vi "Periodic Tasks.vi"(8 "error in":errorcluster) -> ()   [LabVIEW 2018]
doc: "This VI runs in parallel to other tasks. It can contain as many user-defined periodic loops as you need. These can carry out PID or other sorts of timed response."
uses:
  <vilib>/Rock Robotics/WPI/Solenoid/WPI_SolenoidValue.ctl
  <vilib>/Rock Robotics/WPI/ThirdParty/Phoenix-LabVIEW/Motor Controller/Controls/CTRE_Phoenix_MotorControl_ControlMode.ctl
  <vilib>/Rock Robotics/WPI/Utilities/WPI_GetSetVariantRefNum.vi
  Robot Global Data.vi
  <vilib>/Rock Robotics/Network Tables/NT Write Boolean.vi
  <vilib>/Rock Robotics/WPI/ThirdParty/Phoenix-LabVIEW/Motor Controller/Get/CTRE_Phoenix_MotorController_GetSelectedSensorData.vi
  <vilib>/Rock Robotics/Network Tables/NT Write Number.vi
  <vilib>/Rock Robotics/WPI/ThirdParty/Phoenix-LabVIEW/Motor Controller/Get/CTRE_Phoenix_MotorController_GetGeneralStatus.vi
  <vilib>/Rock Robotics/WPI/ThirdParty/Phoenix-LabVIEW/Motor Controller/Get/CTRE_Phoenix_MotorController_GetOutputCurrent_Enhanced.vi
  <vilib>/Rock Robotics/WPI/Solenoid/WPI_SolenoidSetEnum.vi
  Intake Constants.vi
  Elevator Constants.vi
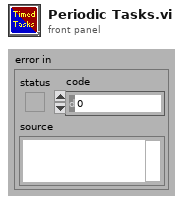
[diagram p1: front panel]
types:
  T1 = enum16{"Zero Power", "Push Cargo", "Pull Cargo", "Hold Cargo"}
  T2 = enum16{"In Up Position", "Seek Up Stage 1", "Seek Up Stage 2", "Seek Normally", "Test Enabled"}
  T3 = typedef "WPI_MotorControlDeviceRef.ctl" = cluster{"DeviceStatus":errorcluster, "Type":T4, "PWM":cluster{"PWM Channel":T5, "DeadBand":T6}, "CAN":cluster{"Device Number":u8, "SetOutput VI Ref":variant, "GetOutput VI Ref":variant, "Enable VI Ref":variant, "Disable VI Ref":variant, "Data":variant}, "Invert":bool, "DIO PWM":cluster{"PWM \"Enable\" Channel":T5, "DIOChannel":T7, "PWM Rate":dbl}}
  T4 = typedef "WPI_MotorControlType.ctl" = enum16{"PWM", "CAN", "DIO PWM"}
  T5 = typedef "FPGA_DIOPWMChannel.ctl" = enum8{"PWM 0", "PWM 1", "PWM 2", "PWM 3", "PWM 4", "PWM 5", "PWM 6", "PWM 7", "PWM 8", "PWM 9", "PWM MXP 0", "PWM MXP 1", "PWM MXP 2", "PWM MXP 3", "PWM MXP 4", "PWM MXP 5", "PWM MXP 6", "PWM MXP 7", "PWM MXP 8", "PWM MXP 9", "Invalid"}
  T6 = typedef "WPI_PWMDeadband.ctl" = cluster{"Name":string, "maxPositivePwm":i32, "minPositivePwm":i32, "centerPwm":i32, "maxNegativePwm":i32, "minNegativePwm":i32, "angularRange":u16}
  T7 = typedef "FPGA_DIOChannel.ctl" = enum8{"DIO 0", "DIO 1", "DIO 2", "DIO 3", "DIO 4", "DIO 5", "DIO 6", "DIO 7", "DIO 8", "DIO 9", "DIO MXP 0", "DIO MXP 1", "DIO MXP 2", "DIO MXP 3", "DIO MXP 4", "DIO MXP 5", "DIO MXP 6", "DIO MXP 7", "DIO MXP 8", "DIO MXP 9", "DIO MXP 10", "DIO MXP 11", "DIO MXP 12", "DIO MXP 13", "DIO MXP 14", "DIO MXP 15", "SPI Port CS1", "SPI Port CS2", "SPI Port CS3", "SPI Port MISO", "SPI Port MOSI", "Invalid"}
  T8 = typedef "WPI_JoystickDevRef.ctl" = cluster{"Device":T9}
  T9 = typedef "WPI_JoystickDeviceEnum.ctl" = enum16{"USB 0", "USB 1", "USB 2", "USB 3", "USB 4", "USB 5"}
  T10 = typedef "WPI_RobotDriveDevRef.ctl" = cluster{"DevStatus":errorcluster, "Motors[]":T3[], "Square Inputs":bool, "Max Output":dbl}
  T11 = typedef "WPI_SolenoidDevRef.ctl" = cluster{"DevStatus":errorcluster, "Pneumatics Control Module":u8, "Forward Solenoid Channel":T12, "Reverse Solenoid Channel":T12}
  T12 = typedef "WPI_SolenoidChannel.ctl" = enum8{"Solenoid 0", "Solenoid 1", "Solenoid 2", "Solenoid 3", "Solenoid 4", "Solenoid 5", "Solenoid 6", "Solenoid 7", "Invalid"}
  T13 = typedef "WPI_CompressorDevRef.ctl" = cluster{"DevStatus":errorcluster, "Pneumatics Control Module":u8}
  T14 = cluster{"PhoenixMotorControlDevRef":T3, "PhoenixMotorControlDevRef":T3, "PhoenixMotorControlDevRef":T3}
  T15 = cluster{"JoystickDevRef":T8, "RobotDriveDevRef":T10, "SolenoidDevRef":T11, "SolenoidDevRef":T11, "CompressorDevRef":T13, "JoystickDevRef":T8}
  T16 = typedef "CTRE_Phoenix_MotorControl_ControlMode.ctl" = u16
  T17 = typedef "WPI_SolenoidValue.ctl" = enum16{"Off", "On", "Forward", "Reverse"}
  T18 = enum16{"In Up Position", "Seek Up Stage 1", "Seek Up Stage 2", "Seek Normally"}
  T19 = typedef "WPI_DriverStationRobotMode2.ctl" = enum16{"Autonomous Disabled", "Autonomous Enabled", "Teleop Disabled", "Teleop Enabled", "Disconnected", "Finish", "Test Disabled", "Test Enabled", "Emergency Stopped"}
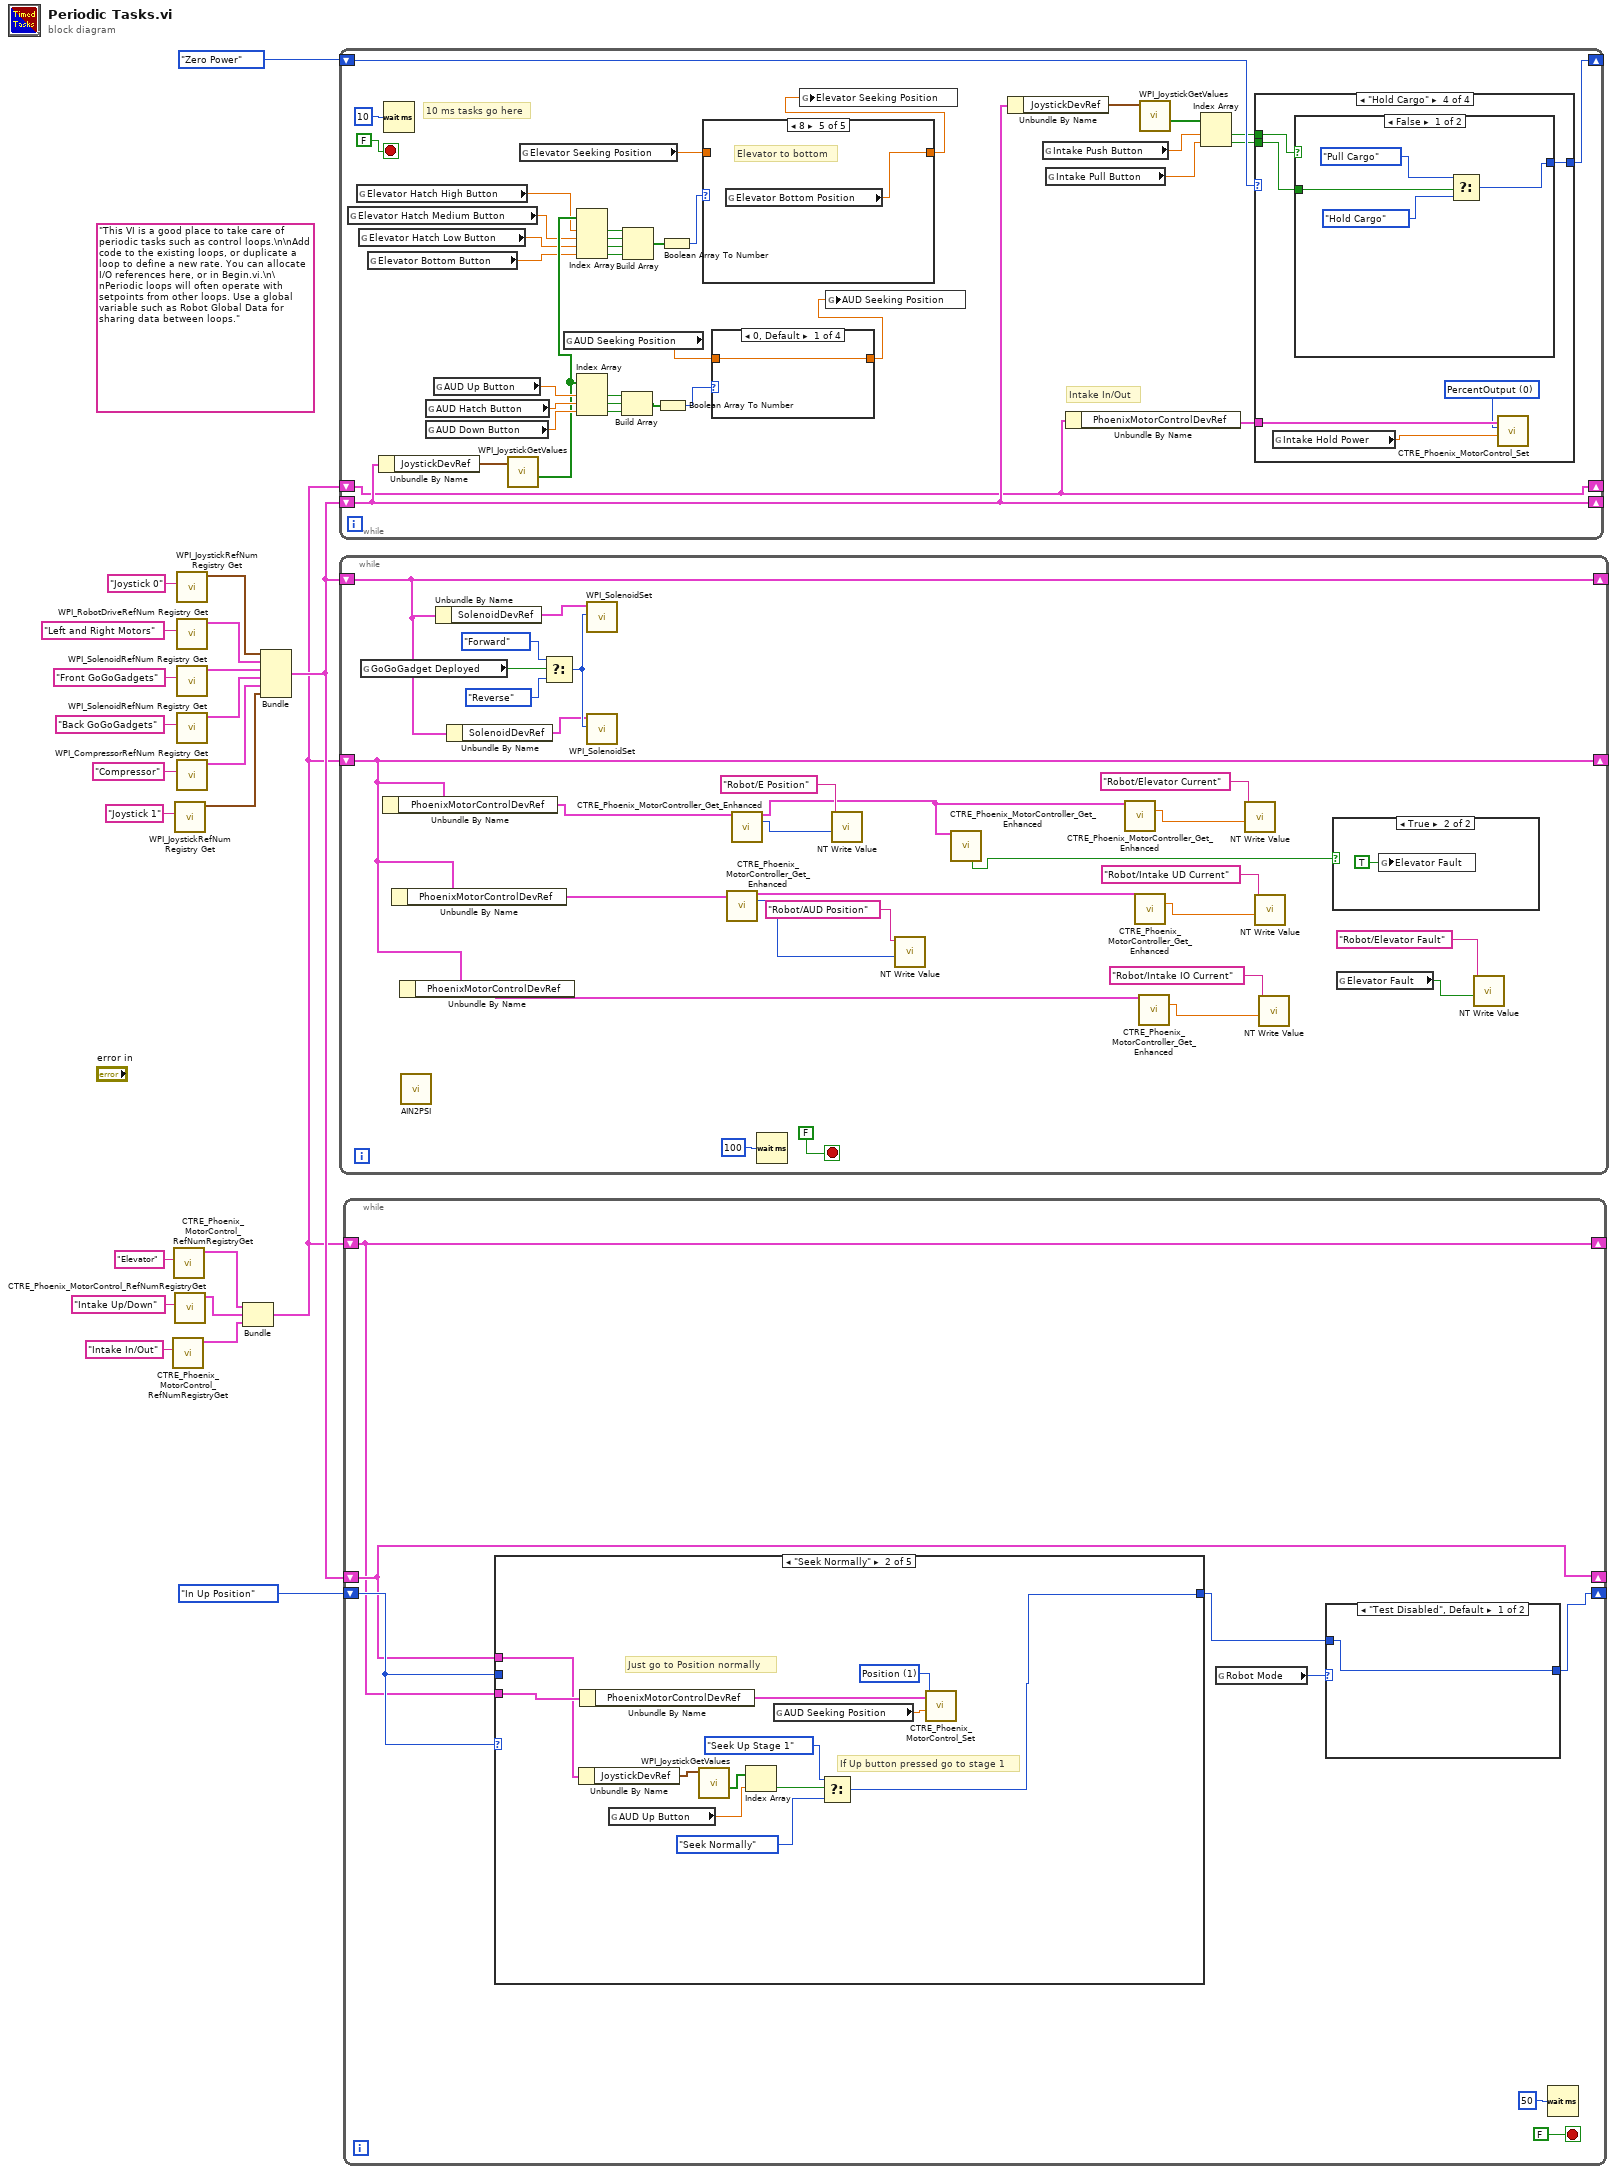
[diagram p0: block diagram]
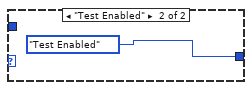
[diagram p2: hidden frame]
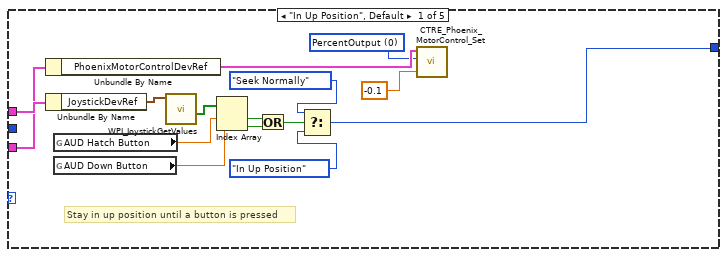
[diagram p3: hidden frame]
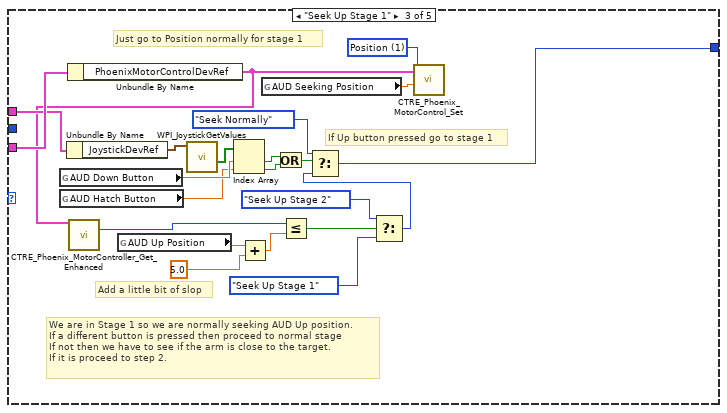
[diagram p4: hidden frame]
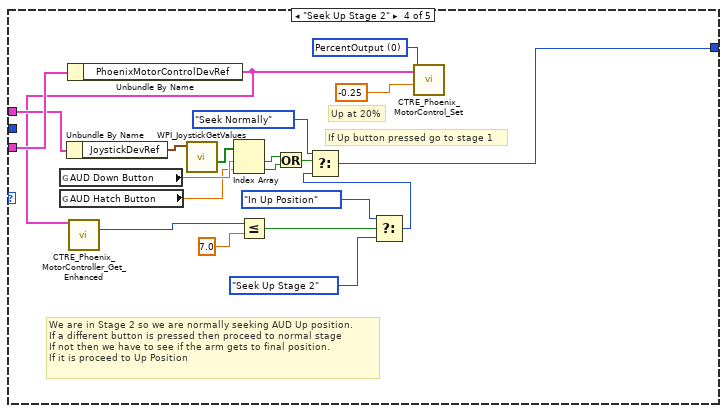
[diagram p5: hidden frame]
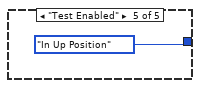
[diagram p6: hidden frame]
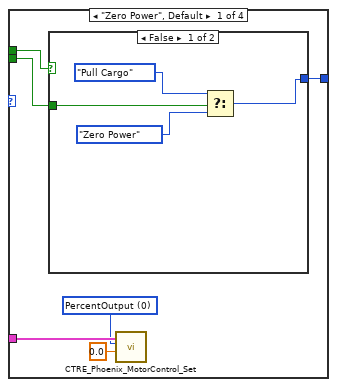
[diagram p8: hidden frame]
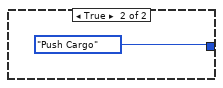
[diagram p9: hidden frame]
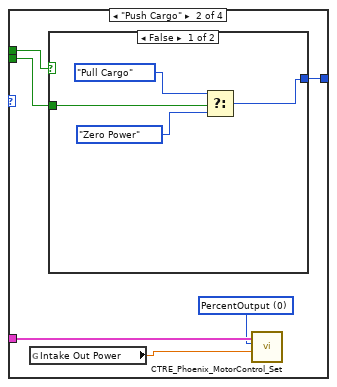
[diagram p10: hidden frame]
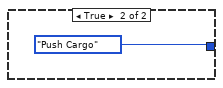
[diagram p11: hidden frame]
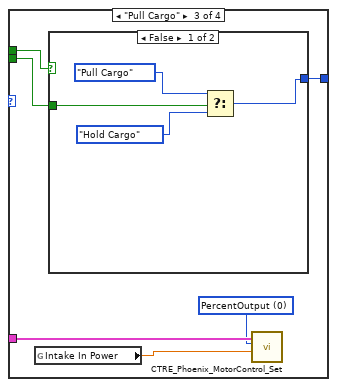
[diagram p12: hidden frame]
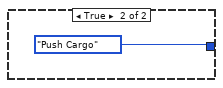
[diagram p13: hidden frame]
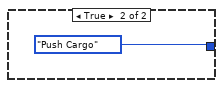
[diagram p14: hidden frame]
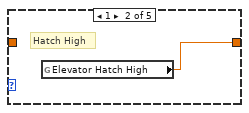
[diagram p16: hidden frame]
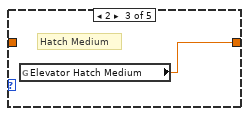
[diagram p17: hidden frame]
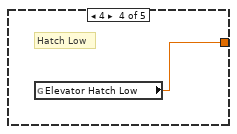
[diagram p18: hidden frame]
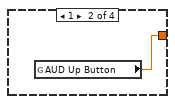
[diagram p19: hidden frame]
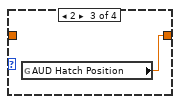
[diagram p20: hidden frame]
diagram:
  (unwired) "This VI is a good place to take care of periodic tasks such as control loops.\n\nAdd code to the existing loops, or duplicate a loop to define a new rate. You can allocate I/O references here, or in Begin.vi.\n\nPeriodic loops will often operate with setpoints from other loops. Use a global variable such as Robot Global Data for sharing data between loops."
  n1 = call <vilib>:"CTRE_Phoenix_MotorControl_RefNumRegistryGet.vi"("refnum name"="Intake In/Out") -> ("PhoenixMotorControlDevRef"=w7:T3)  [unwired: 9 in, 1 out]
  n2 = call <vilib>:"CTRE_Phoenix_MotorControl_RefNumRegistryGet.vi"("refnum name"="Elevator") -> ("PhoenixMotorControlDevRef"=w5:T3)  [unwired: 9 in, 1 out]
  n3 = call <vilib>:"WPI_JoystickRefNum Registry Get.vi"("refnum name"="Joystick 1") -> ("JoystickDevRef"=w11:T8)  [unwired: 1 in, 9 out]
  n4 = call <vilib>:"CTRE_Phoenix_MotorControl_RefNumRegistryGet.vi"("refnum name"="Intake Up/Down") -> ("PhoenixMotorControlDevRef"=w6:T3)  [unwired: 9 in, 1 out]
  n5 = call <vilib>:"WPI_JoystickRefNum Registry Get.vi"("refnum name"="Joystick 0") -> ("JoystickDevRef"=w20:T8)  [unwired: 1 in, 9 out]
  n6 = call <vilib>:"WPI_RobotDriveRefNum Registry Get.vi"("refnum name"="Left and Right Motors") -> ("RobotDriveDevRef"=w19:T10)  [unwired: 1 in, 9 out]
  n7 = call <vilib>:"WPI_SolenoidRefNum Registry Get.vi"("refnum name"="Front GoGoGadgets") -> ("SolenoidDevRef"=w18:T11)  [unwired: 9 in, 1 out]
  n8 = call <vilib>:"WPI_SolenoidRefNum Registry Get.vi"("refnum name"="Back GoGoGadgets") -> ("SolenoidDevRef"=w17:T11)  [unwired: 9 in, 1 out]
  n9 = call <vilib>:"WPI_CompressorRefNum Registry Get.vi"("refnum name"="Compressor") -> ("CompressorDevRef"=w13:T13)  [unwired: 9 in, 1 out]
  n10 = Bundle("PhoenixMotorControlDevRef"=w5, "PhoenixMotorControlDevRef"=w6, "PhoenixMotorControlDevRef"=w7) -> (w1:T14)  [unwired: 1 in]
  n11 = Bundle("JoystickDevRef"=w20, "RobotDriveDevRef"=w19, "SolenoidDevRef"=w18, "SolenoidDevRef"=w17, "CompressorDevRef"=w13, "JoystickDevRef"=w11) -> (w3:T15)  [unwired: 1 out]
  n12 = while {
    shift-right: [w32] -> _
    shift-left: w3 -> [w32]
    shift-right: [w23] -> _
    shift-left: T1."Zero Power" -> [w28]
    shift-right: [w27] -> _
    shift-left: w1 -> [w27]
    stop <- FALSE stop-if-true
    # "Intake In/Out"
    # "10 ms tasks go here"
    n13 = global read "Elevator Constants.vi" "Elevator Hatch Medium Button"() -> (w43:dbl)
    n14 = global read "Elevator Constants.vi" "Elevator Hatch High Button"() -> (w42:dbl)
    n15 = global read "Elevator Constants.vi" "Elevator Hatch Low Button"() -> (w44:dbl)
    n16 = global read "Elevator Constants.vi" "Elevator Bottom Button"() -> (w45:dbl)
    n17 = Unbundle By Name(w32) -> ("JoystickDevRef"=w57:T8)
    n18 = Wait (ms)(milliseconds to wait=u32 10) -> ()  [unwired: 1 out]
    n19 = global read "Intake Constants.vi" "AUD Hatch Button"() -> (w55:dbl)
    n20 = global read "Intake Constants.vi" "AUD Down Button"() -> (w51:dbl)
    n21 = global read "Intake Constants.vi" "AUD Up Button"() -> (w56:dbl)
    n22 = call <vilib>:"WPI_JoystickGetValues.vi"("JoystickDevRef"=w57) -> ("Buttons"=w46:bool[])  [unwired: 6 in, 4 out]
    n23 = global read "Elevator Constants.vi" "Elevator Seeking Position"() -> (w35:dbl)
    n24 = global read "Intake Constants.vi" "AUD Seeking Position"() -> (w49:dbl)
    n25 = Index Array(array=w46, index #1=w42, index #2=w43, index #3=w44, index #4=w45) -> (element #1=w38:bool, element #2=w41:bool, element #3=w39:bool, element #4=w40:bool)
    n26 = Index Array(array=w46, index #1=w56, index #2=w55, index #3=w51) -> (element #1=w54:bool, element #2=w53:bool, element #3=w52:bool)
    n27 = Build Array(w54, w53, w52) -> (w50:bool[])
    n28 = Build Array(w38, w41, w39, w40) -> (w37:bool[])
    n29 = Boolean Array To Number(Boolean array=w50) -> (number=w48:u32)
    n30 = Boolean Array To Number(Boolean array=w37) -> (number=w36:u32)
    n31 = case shown="8" w36 {
      tunnel: w35 -> [w104 _ _ _ _]
      tunnel: [w104 w105 w106 w107 w108] -> w34
      frame 0, Default {
      }
      frame 1 {
        # "Hatch High"
        n32 = global read "Elevator Constants.vi" "Elevator Hatch High"() -> (w105:dbl)
      }
      frame 2 {
        # "Hatch Medium"
        n33 = global read "Elevator Constants.vi" "Elevator Hatch Medium"() -> (w106:dbl)
      }
      frame 4 {
        # "Hatch Low"
        n34 = global read "Elevator Constants.vi" "Elevator Hatch Low"() -> (w107:dbl)
      }
      frame 8 {
        # "Elevator to bottom"
        n35 = global read "Elevator Constants.vi" "Elevator Bottom Position"() -> (w108:dbl)
      }
    }
    n36 = case shown="0, Default" w48 {
      tunnel: w49 -> [w109 _ _ _]
      tunnel: [w109 w110 w111 w112] -> w47
      frame 0, Default {
      }
      frame 1 {
        n37 = global read "Intake Constants.vi" "AUD Up Button"() -> (w110:dbl)
      }
      frame 2 {
        n38 = global read "Intake Constants.vi" "AUD Hatch Position"() -> (w111:dbl)
      }
      frame 4 {
        n39 = global read "Intake Constants.vi" "AUD Down Position"() -> (w112:dbl)
      }
    }
    n40 = global write "Elevator Constants.vi" "Elevator Seeking Position"(w34) -> ()
    n41 = global write "Intake Constants.vi" "AUD Seeking Position"(w47) -> ()
    n42 = Unbundle By Name(w32) -> ("JoystickDevRef"=w33:T8)
    n43 = global read "Intake Constants.vi" "Intake Push Button"() -> (w30:dbl)
    n44 = global read "Intake Constants.vi" "Intake Pull Button"() -> (w29:dbl)
    n45 = Unbundle By Name(w27) -> ("PhoenixMotorControlDevRef"=w26:T3)
    n46 = call <vilib>:"WPI_JoystickGetValues.vi"("JoystickDevRef"=w33) -> ("Buttons"=w31:bool[])  [unwired: 6 in, 4 out]
    n47 = Index Array(array=w31, index #1=w30, index #2=w29) -> (element #1=w25:bool, element #2=w24:bool)
    n48 = case shown="\"Hold Cargo\"" w28 {
      tunnel: w26 -> [w65 w76 w87 w98]
      tunnel: w25 -> [w62 w74 w85 w96]
      tunnel: w24 -> [w61 w73 w84 w95]
      tunnel: [w60 w72 w83 w94] -> w23
      frame "Zero Power", Default {
        w64 = T16 0 items=["PercentOutput"=0, "Position"=1, "Velocity"=2, "Current"=3, "Follower"=5, "MotionProfile"=6, "MotionMagic"=7, "MotionProfileArc"=10, "Disabled"=15] ("Control Mode")
        n49 = case shown="False" w62 {
          tunnel: w61 -> [w69 _]
          tunnel: [w66 T1."Push Cargo"] -> w60
          frame False {
            n50 = Select(t=T1."Pull Cargo", s=w69, f=T1."Zero Power") -> (s? t:f=w66:T1)
          }
          frame True {
          }
        }
        n51 = call <vilib>:"CTRE_Phoenix_MotorControl_Set.vi"("Output"=0.0, "Control Mode"=w64, "PhoenixMotorControlDevRef"=w65) -> ()  [unwired: 7 in, 2 out]
      }
      frame "Push Cargo" {
        w75 = T16 0 items=["PercentOutput"=0, "Position"=1, "Velocity"=2, "Current"=3, "Follower"=5, "MotionProfile"=6, "MotionMagic"=7, "MotionProfileArc"=10, "Disabled"=15] ("Control Mode")
        n52 = global read "Intake Constants.vi" "Intake Out Power"() -> (w71:dbl)
        n53 = case shown="False" w74 {
          tunnel: w73 -> [w80 _]
          tunnel: [w77 T1."Push Cargo"] -> w72
          frame False {
            n54 = Select(t=T1."Pull Cargo", s=w80, f=T1."Zero Power") -> (s? t:f=w77:T1)
          }
          frame True {
          }
        }
        n55 = call <vilib>:"CTRE_Phoenix_MotorControl_Set.vi"("Output"=w71, "Control Mode"=w75, "PhoenixMotorControlDevRef"=w76) -> ()  [unwired: 7 in, 2 out]
      }
      frame "Pull Cargo" {
        w86 = T16 0 items=["PercentOutput"=0, "Position"=1, "Velocity"=2, "Current"=3, "Follower"=5, "MotionProfile"=6, "MotionMagic"=7, "MotionProfileArc"=10, "Disabled"=15] ("Control Mode")
        n56 = global read "Intake Constants.vi" "Intake In Power"() -> (w82:dbl)
        n57 = case shown="False" w85 {
          tunnel: w84 -> [w91 _]
          tunnel: [w88 T1."Push Cargo"] -> w83
          frame False {
            n58 = Select(t=T1."Pull Cargo", s=w91, f=T1."Hold Cargo") -> (s? t:f=w88:T1)
          }
          frame True {
          }
        }
        n59 = call <vilib>:"CTRE_Phoenix_MotorControl_Set.vi"("Output"=w82, "Control Mode"=w86, "PhoenixMotorControlDevRef"=w87) -> ()  [unwired: 7 in, 2 out]
      }
      frame "Hold Cargo" {
        w97 = T16 0 items=["PercentOutput"=0, "Position"=1, "Velocity"=2, "Current"=3, "Follower"=5, "MotionProfile"=6, "MotionMagic"=7, "MotionProfileArc"=10, "Disabled"=15] ("Control Mode")
        n60 = global read "Intake Constants.vi" "Intake Hold Power"() -> (w93:dbl)
        n61 = case shown="False" w96 {
          tunnel: w95 -> [w102 _]
          tunnel: [w99 T1."Push Cargo"] -> w94
          frame False {
            n62 = Select(t=T1."Pull Cargo", s=w102, f=T1."Hold Cargo") -> (s? t:f=w99:T1)
          }
          frame True {
          }
        }
        n63 = call <vilib>:"CTRE_Phoenix_MotorControl_Set.vi"("Output"=w93, "Control Mode"=w97, "PhoenixMotorControlDevRef"=w98) -> ()  [unwired: 7 in, 2 out]
      }
    }
  }
  n64 = while {
    shift-right: [w132] -> _
    shift-left: w3 -> [w132]
    shift-right: [w117] -> _
    shift-left: w1 -> [w117]
    stop <- FALSE stop-if-true
    n65 = global read "Robot Global Data.vi" "GoGoGadget Deployed"() -> (w135:bool)
    n66 = Unbundle By Name(w117) -> ("PhoenixMotorControlDevRef"=w124:T3)
    n67 = Unbundle By Name(w117) -> ("PhoenixMotorControlDevRef"=w123:T3)
    n68 = Unbundle By Name(w117) -> ("PhoenixMotorControlDevRef"=w127:T3)
    n69 = call "AIN2PSI.vi"() -> ()  [unwired: 11 in, 1 out]
    n70 = Unbundle By Name(w132) -> ("SolenoidDevRef"=w134:T11)
    n71 = Unbundle By Name(w132) -> ("SolenoidDevRef"=w133:T11)
    n72 = Select(t=WPI_SolenoidValue."Forward" ("Value"), s=w135, f=WPI_SolenoidValue."Reverse") -> (s? t:f=w138:T17)
    n73 = call-poly <vilib>:"WPI_SolenoidSet.vi"("Value"=w138, "SolenoidDevRef"=w134) -> ()  [unwired: 8 in, 2 out]
    n74 = call-poly <vilib>:"WPI_SolenoidSet.vi"("Value"=w138, "SolenoidDevRef"=w133) -> ()  [unwired: 8 in, 2 out]
    n75 = call-poly <vilib>:"CTRE_Phoenix_MotorController_Get_Enhanced.vi"("PhoenixMotorControlDevRef"=w123) -> ("PhoenixMotorControlDevRef"=w122:T3, "Position (Raw Sensor Units)"=w118:i32)  [unwired: 11 in, 2 out]
    n76 = call-poly <vilib>:"CTRE_Phoenix_MotorController_Get_Enhanced.vi"("PhoenixMotorControlDevRef"=w124) -> ("PhoenixMotorControlDevRef"=w116:T3, "Position (Raw Sensor Units)"=w119:i32)  [unwired: 11 in, 2 out]
    n77 = Wait (ms)(milliseconds to wait=u32 100) -> ()  [unwired: 1 out]
    n78 = call-poly <vilib>:"NT Write Value.vi"("Numeric"=w119, "Name"="Robot/E Position") -> ()  [unwired: 9 in, 1 out]
    n79 = call-poly <vilib>:"NT Write Value.vi"("Numeric"=w118, "Name"="Robot/AUD Position") -> ()  [unwired: 9 in, 1 out]
    n80 = call-poly <vilib>:"CTRE_Phoenix_MotorController_Get_Enhanced.vi"("PhoenixMotorControlDevRef"=w116) -> ("Has Reset Occurred?"=w115:bool)  [unwired: 9 in, 5 out]
    n81 = call-poly <vilib>:"CTRE_Phoenix_MotorController_Get_Enhanced.vi"("PhoenixMotorControlDevRef"=w116) -> ("Output Current"=w130:dbl)  [unwired: 12 in, 2 out]
    n82 = call-poly <vilib>:"CTRE_Phoenix_MotorController_Get_Enhanced.vi"("PhoenixMotorControlDevRef"=w122) -> ("Output Current"=w129:dbl)  [unwired: 12 in, 2 out]
    n83 = call-poly <vilib>:"CTRE_Phoenix_MotorController_Get_Enhanced.vi"("PhoenixMotorControlDevRef"=w127) -> ("Output Current"=w125:dbl)  [unwired: 12 in, 2 out]
    n84 = call-poly <vilib>:"NT Write Value.vi"("Numeric"=w130, "Name"="Robot/Elevator Current") -> ()  [unwired: 9 in, 1 out]
    n85 = call-poly <vilib>:"NT Write Value.vi"("Numeric"=w129, "Name"="Robot/Intake UD Current") -> ()  [unwired: 9 in, 1 out]
    n86 = call-poly <vilib>:"NT Write Value.vi"("Numeric"=w125, "Name"="Robot/Intake IO Current") -> ()  [unwired: 9 in, 1 out]
    n87 = case shown="True" w115 {
      frame False {
      }
      frame True {
        n88 = global write "Robot Global Data.vi" "Elevator Fault"(TRUE ("Elevator Fault")) -> ()
      }
    }
    n89 = global read "Robot Global Data.vi" "Elevator Fault"() -> (w114:bool)
    n90 = call-poly <vilib>:"NT Write Value.vi"("Boolean"=w114, "Name"="Robot/Elevator Fault") -> ()  [unwired: 9 in, 1 out]
  }
  n91 = while {
    shift-right: [w142] -> _
    shift-left: w1 -> [w142]
    shift-right: [w143] -> _
    shift-left: T2."In Up Position" -> [w147]
    shift-right: [w146] -> _
    shift-left: w3 -> [w146]
    stop <- FALSE stop-if-true
    n92 = case shown="\"Seek Normally\"" w147 {
      tunnel: w147 -> [_ _ _ _ _]
      tunnel: w146 -> [w166 w173 w196 w217 _]
      tunnel: w142 -> [w165 w178 w200 w220 _]
      tunnel: [w156 w167 w192 w213 T2."In Up Position"] -> w144
      frame "In Up Position", Default {
        w153 = T16 0 items=["PercentOutput"=0, "Position"=1, "Velocity"=2, "Current"=3, "Follower"=5, "MotionProfile"=6, "MotionMagic"=7, "MotionProfileArc"=10, "Disabled"=15] ("Control Mode")
        # "Stay in up position until a button is pressed"
        n93 = Unbundle By Name(w165) -> ("PhoenixMotorControlDevRef"=w154:T3)
        n94 = Unbundle By Name(w166) -> ("JoystickDevRef"=w164:T8)
        n95 = global read "Intake Constants.vi" "AUD Hatch Button"() -> (w163:dbl)
        n96 = global read "Intake Constants.vi" "AUD Down Button"() -> (w162:dbl)
        n97 = call <vilib>:"WPI_JoystickGetValues.vi"("JoystickDevRef"=w164) -> ("Buttons"=w158:bool[])  [unwired: 6 in, 4 out]
        n98 = Index Array(array=w158, index #1=w163, index #2=w162) -> (element #1=w160:bool, element #2=w161:bool)
        n99 = Or(x=w160, y=w161) -> (x .or. y?=w159:bool)
        n100 = Select(t=T18."Seek Normally", s=w159, f=T18."In Up Position") -> (s? t:f=w156:T18)
        n101 = call <vilib>:"CTRE_Phoenix_MotorControl_Set.vi"("Output"=-0.1, "Control Mode"=w153, "PhoenixMotorControlDevRef"=w154) -> ()  [unwired: 7 in, 2 out]
      }
      frame "Seek Normally" {
        w177 = T16 1 items=["PercentOutput"=0, "Position"=1, "Velocity"=2, "Current"=3, "Follower"=5, "MotionProfile"=6, "MotionMagic"=7, "MotionProfileArc"=10, "Disabled"=15] ("Control Mode")
        # "If Up button pressed go to stage 1"
        # "Just go to Position normally"
        n102 = Unbundle By Name(w173) -> ("JoystickDevRef"=w174:T8)
        n103 = Unbundle By Name(w178) -> ("PhoenixMotorControlDevRef"=w175:T3)
        n104 = global read "Intake Constants.vi" "AUD Up Button"() -> (w171:dbl)
        n105 = call <vilib>:"WPI_JoystickGetValues.vi"("JoystickDevRef"=w174) -> ("Buttons"=w172:bool[])  [unwired: 6 in, 4 out]
        n106 = Index Array(array=w172, index=w171) -> (element=w169:bool)
        n107 = global read "Intake Constants.vi" "AUD Seeking Position"() -> (w176:dbl)
        n108 = Select(t=T18."Seek Up Stage 1", s=w169, f=T18."Seek Normally") -> (s? t:f=w167:T18)
        n109 = call <vilib>:"CTRE_Phoenix_MotorControl_Set.vi"("Output"=w176, "Control Mode"=w177, "PhoenixMotorControlDevRef"=w175) -> ()  [unwired: 7 in, 2 out]
      }
      frame "Seek Up Stage 1" {
        w199 = T16 1 items=["PercentOutput"=0, "Position"=1, "Velocity"=2, "Current"=3, "Follower"=5, "MotionProfile"=6, "MotionMagic"=7, "MotionProfileArc"=10, "Disabled"=15] ("Control Mode")
        # "We are in Stage 1 so we are normally seeking AUD Up position.\nIf a different button is pressed then proceed to normal stage\nIf not then we have to see if the arm is close to the target.\nIf it is proceed to step 2."
        # "Add a little bit of slop"
        # "If Up button pressed go to stage 1"
        # "Just go to Position normally for stage 1"
        n110 = global read "Intake Constants.vi" "AUD Down Button"() -> (w194:dbl)
        n111 = global read "Intake Constants.vi" "AUD Hatch Button"() -> (w191:dbl)
        n112 = Unbundle By Name(w196) -> ("JoystickDevRef"=w197:T8)
        n113 = Unbundle By Name(w200) -> ("PhoenixMotorControlDevRef"=w187:T3)
        n114 = call-poly <vilib>:"CTRE_Phoenix_MotorController_Get_Enhanced.vi"("PhoenixMotorControlDevRef"=w187) -> ("Position (Raw Sensor Units)"=w186:i32)  [unwired: 11 in, 3 out]
        n115 = global read "Intake Constants.vi" "AUD Up Position"() -> (w185:dbl)
        n116 = call <vilib>:"WPI_JoystickGetValues.vi"("JoystickDevRef"=w197) -> ("Buttons"=w195:bool[])  [unwired: 6 in, 4 out]
        n117 = Index Array(array=w195, index #1=w194, index #2=w191) -> (element #1=w190:bool, element #2=w189:bool)
        n118 = Add(x=w185, y=5.0) -> (x+y=w183:dbl)
        n119 = global read "Intake Constants.vi" "AUD Seeking Position"() -> (w198:dbl)
        n120 = Or(x=w190, y=w189) -> (x .or. y?=w188:bool)
        n121 = Less Or Equal?(x=w186, y=w183) -> (x <= y?=w182:bool)
        n122 = Select(t=T18."Seek Up Stage 2", s=w182, f=T18."Seek Up Stage 1") -> (s? t:f=w179:T18)
        n123 = Select(t=T18."Seek Normally", s=w188, f=w179) -> (s? t:f=w192:T18)
        n124 = call <vilib>:"CTRE_Phoenix_MotorControl_Set.vi"("Output"=w198, "Control Mode"=w199, "PhoenixMotorControlDevRef"=w187) -> ()  [unwired: 7 in, 2 out]
      }
      frame "Seek Up Stage 2" {
        w219 = T16 0 items=["PercentOutput"=0, "Position"=1, "Velocity"=2, "Current"=3, "Follower"=5, "MotionProfile"=6, "MotionMagic"=7, "MotionProfileArc"=10, "Disabled"=15] ("Control Mode")
        # "Up at 20%"
        # "We are in Stage 2 so we are normally seeking AUD Up position.\nIf a different button is pressed then proceed to normal stage\nIf not then we have to see if the arm gets to final position.\nIf it is proceed to Up Position"
        # "If Up button pressed go to stage 1"
        n125 = global read "Intake Constants.vi" "AUD Down Button"() -> (w215:dbl)
        n126 = global read "Intake Constants.vi" "AUD Hatch Button"() -> (w212:dbl)
        n127 = Unbundle By Name(w217) -> ("JoystickDevRef"=w218:T8)
        n128 = Unbundle By Name(w220) -> ("PhoenixMotorControlDevRef"=w208:T3)
        n129 = call-poly <vilib>:"CTRE_Phoenix_MotorController_Get_Enhanced.vi"("PhoenixMotorControlDevRef"=w208) -> ("Position (Raw Sensor Units)"=w207:i32)  [unwired: 11 in, 3 out]
        n130 = call <vilib>:"WPI_JoystickGetValues.vi"("JoystickDevRef"=w218) -> ("Buttons"=w216:bool[])  [unwired: 6 in, 4 out]
        n131 = Index Array(array=w216, index #1=w215, index #2=w212) -> (element #1=w211:bool, element #2=w210:bool)
        n132 = Less Or Equal?(x=w207, y=7.0) -> (x <= y?=w206:bool)
        n133 = Or(x=w211, y=w210) -> (x .or. y?=w209:bool)
        n134 = Select(t=T18."In Up Position", s=w206, f=T18."Seek Up Stage 2") -> (s? t:f=w203:T18)
        n135 = Select(t=T18."Seek Normally", s=w209, f=w203) -> (s? t:f=w213:T18)
        n136 = call <vilib>:"CTRE_Phoenix_MotorControl_Set.vi"("Output"=-0.25, "Control Mode"=w219, "PhoenixMotorControlDevRef"=w208) -> ()  [unwired: 7 in, 2 out]
      }
      frame "Test Enabled" {
      }
    }
    n137 = global read "Robot Global Data.vi" "Robot Mode"() -> (w145:T19)
    n138 = case shown="\"Test Disabled\", Default" w145 {
      tunnel: w144 -> [w150 _]
      tunnel: [w150 T2."Test Enabled"] -> w143
      frame "Test Disabled", Default {
      }
      frame "Test Enabled" {
      }
    }
    n139 = Wait (ms)(milliseconds to wait=u32 50) -> ()  [unwired: 1 out]
  }
